vi "Run Command-Chris 1.9.vi"(2 "Line Index In":i32, 3 "Script":string) -> (0 "Line Index Out":i32, 1 "Done":bool)   [LabVIEW 2017, in "Apple script.lvlib"]
doc: "Looks at a line and runs the appropriate command. Add new commands to this vi."
uses:
  Apple script.lvlib
  Robot Global Data.vi
  <vilib>/addons/control/pid/pid.llb/PID.vi
  <vilib>/addons/control/pid/pid.llb/PID (DBL).vi
  Support Code/Angle Distance.vi
  Support Code/Pigeon Gyro.vi
  Support Code/Encoders.vi
  <vilib>/Rock Robotics/Network Tables/NT Write Value.vi
  <vilib>/Rock Robotics/Network Tables/NT Write Numeric Array.vi
  Timer.vi
  Parse Subcommand.vi
panel:
  in  "Error? 2":bool
  in  "Error?":bool
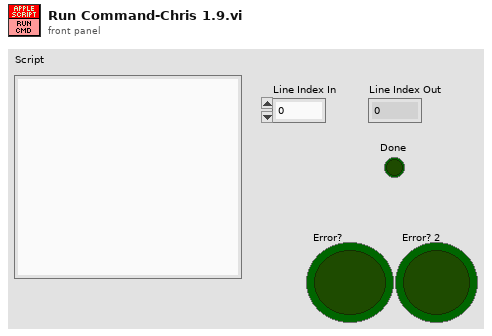
[diagram p1: front panel]
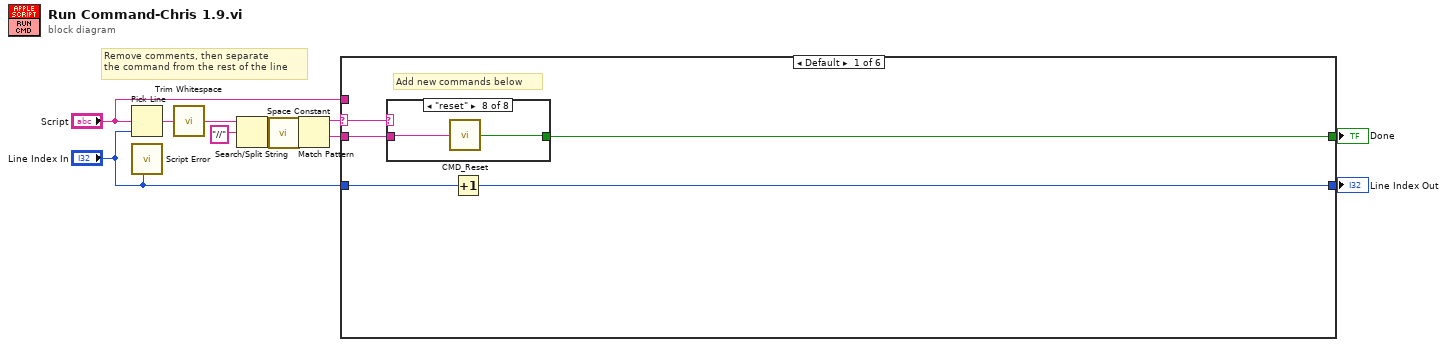
[diagram p0: block diagram]
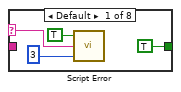
[diagram p2: hidden frame]
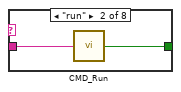
[diagram p3: hidden frame]
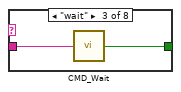
[diagram p4: hidden frame]
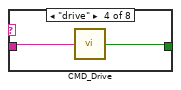
[diagram p5: hidden frame]
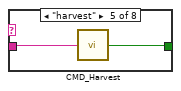
[diagram p6: hidden frame]
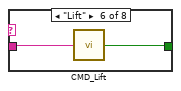
[diagram p7: hidden frame]
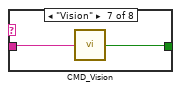
[diagram p8: hidden frame]
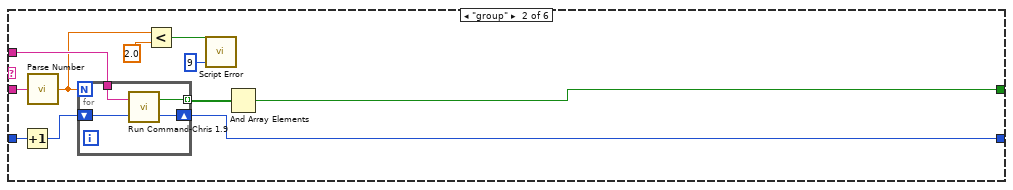
[diagram p9: hidden frame]
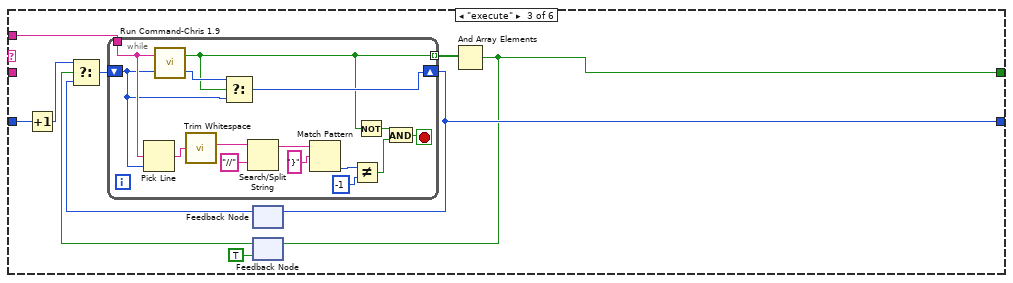
[diagram p10: hidden frame]
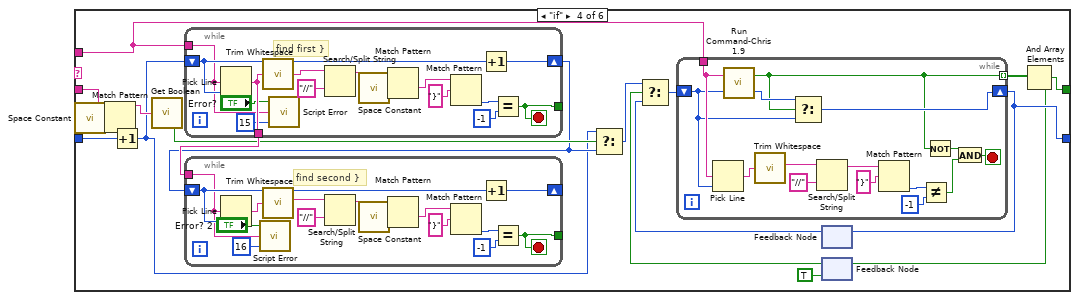
[diagram p11: hidden frame]
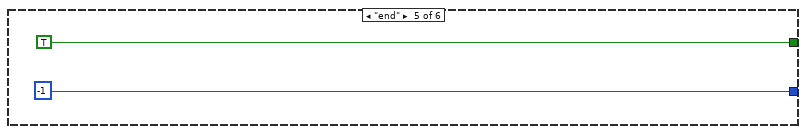
[diagram p12: hidden frame]
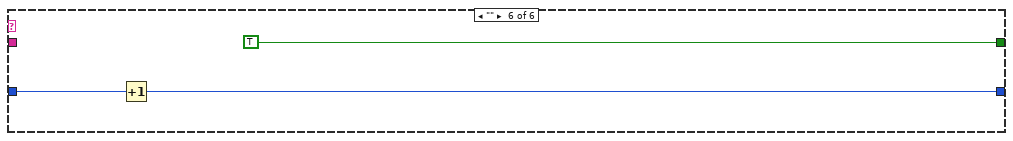
[diagram p13: hidden frame]
diagram:
  # "Remove comments, then separate\nthe command from the rest of the line"
  n1 = Pick Line(multi-line string="Script", line index="Line Index In") -> (output string=w8:string)  [unwired: 1 in]
  n2 = call "Script Error.vi"("Line Number"="Line Index In") -> ()  [unwired: 4 in, 1 out]
  n3 = call <vilib>:"Trim Whitespace.vi"("string"=w8) -> ("trimmed string"=w6:string)  [unwired: 1 in]
  n4 = Search/Split String(string=w6, search string/char (-)="//") -> (substring before match=w5:string)  [unwired: 1 in, 2 out]
  n5 = call <vilib>:"Space Constant.vi"() -> ("String"=w11:string)
  n6 = Match Pattern(string=w5, regular expression=w11) -> (before substring=w4:string, after substring=w3:string)  [unwired: 1 in, 2 out]
  n7 = case shown="Default" w4 {
    selector: w4 -> [w14 _ _ _ _ _]
    tunnel: "Script" -> [_ w45 w58 w83 _ _]
    tunnel: "Line Index In" -> [w16 w43 w59 w77 _ w140]
    tunnel: [w13 w35 w52 w81 TRUE ("Running") TRUE ("Running")] -> w2
    tunnel: [w15 w44 w53 w82 -1 ("Line Index Out") w139] -> w1
    tunnel: w3 -> [w12 w37 _ w78 _ _]
    frame Default {
      # "Add new commands below"
      n8 = case shown="\"reset\"" w14 {
        selector: w14 -> [w17 _ _ _ _ _ _ _]
        tunnel: [TRUE w21 w24 w25 w27 w29 w31 w33] -> w13
        tunnel: w12 -> [_ w22 w23 w26 w28 w30 w32 w34]
        frame Default {
          n9 = call "Script Error.vi"("Error?"=TRUE, "Error Details"=w17, "Error Code"=3) -> ()  [unwired: 2 in, 1 out]
        }
        frame "run" {
          n10 = call "CMD_Run.vi"("Line"=w22) -> ("Done"=w21:bool)
        }
        frame "wait" {
          n11 = call "CMD_Wait.vi"("Line"=w23) -> ("Done"=w24:bool)
        }
        frame "drive" {
          n12 = call "CMD_Drive.vi"("Line"=w26) -> ("Done"=w25:bool)
        }
        frame "harvest" {
          n13 = call "CMD_Harvest.vi"("Line"=w28) -> ("Done"=w27:bool)
        }
        frame "Lift" {
          n14 = call "CMD_Lift.vi"("Line"=w30) -> ("Done"=w29:bool)
        }
        frame "Vision" {
          n15 = call "CMD_Vision.vi"("Line"=w32) -> ("Done"=w31:bool)
        }
        frame "reset" {
          n16 = call "CMD_Reset.vi"("Line"=w34) -> ("Done"=w33:bool)
        }
      }
      n17 = Increment(x=w16) -> (x+1=w15:i32)
    }
    frame "group" {
      n18 = Increment(x=w43) -> (x+1=w42:i32)
      n19 = call "Parse Number.vi"("String"=w37) -> ("Number"=w40:dbl)
      n20 = for {
        N: w40 -> [_]
        tunnel: w45 -> [w49]
        tunnel: [w48] -> w36 mode=indexing
        shift-right: [w47] -> w44
        shift-left: w42 -> [w46]
        n21 = call "Run Command-Chris 1.9.vi"("Line Index In"=w46, "Script"=w49) -> ("Line Index Out"=w47:i32, "Done"=w48:bool)
      }
      n22 = Less?(x=w40, y=2.0) -> (x < y?=w39:bool)
      n23 = call "Script Error.vi"("Error?"=w39, "Error Code"=9) -> ()  [unwired: 3 in, 1 out]
      n24 = And Array Elements(Boolean array=w36) -> (logical AND=w35:bool)
    }
    frame "execute" {
      n25 = Increment(x=w59) -> (x+1=w55:i32)
      n26 = feedback #1() -> (w54:i32)  [unwired: 1 in]
      n27 = feedback #2(TRUE) -> (w51:bool)
      n28 = Select(t=w55, s=w51, f=w54) -> (s? t:f=w56:i32)
      n29 = while {
        tunnel: w58 -> [w68]
        tunnel: [w61] -> w57 mode=indexing
        shift-right: [w65] -> w53
        shift-left: w56 -> [w64]
        stop <- w60 stop-if-true
        n30 = Pick Line(multi-line string=w68, line index=w64) -> (output string=w70:string)  [unwired: 1 in]
        n31 = call "Run Command-Chris 1.9.vi"("Line Index In"=w64, "Script"=w68) -> ("Line Index Out"=w66:i32, "Done"=w61:bool)
        n32 = call <vilib>:"Trim Whitespace.vi"("string"=w70) -> ("trimmed string"=w71:string)  [unwired: 1 in]
        n33 = Select(t=w66, s=w61, f=w64) -> (s? t:f=w65:i32)
        n34 = Search/Split String(string=w71, search string/char (-)="//") -> (substring before match=w67:string)  [unwired: 1 in, 2 out]
        n35 = Match Pattern(string=w67, regular expression="}" ("search string/char (-)")) -> (offset past match=w73:i32)  [unwired: 1 in, 3 out]
        n36 = Not Equal?(x=w73, y=-1) -> (x != y?=w63:bool)
        n37 = Not(x=w61) -> (.not. x?=w62:bool)
        n38 = And(x=w62, y=w63) -> (x .and. y?=w60:bool)
      }
      n39 = feedback-in #1(w53) -> ()
      n40 = And Array Elements(Boolean array=w57) -> (logical AND=w52:bool)
      n41 = feedback-in #2(w52) -> ()
    }
    frame "if" {
      n42 = call <vilib>:"Space Constant.vi"() -> ("String"=w80:string)
      n43 = Match Pattern(string=w78, regular expression=w80) -> (before substring=w79:string)  [unwired: 1 in, 3 out]
      n44 = Increment(x=w77) -> (x+1=w76:i32)
      n45 = call "Get Boolean.vi"("Name"=w79) -> ("Value"=w90:bool)
      n46 = while {
        tunnel: w83 -> [w124]
        shift-right: [w128] -> w89
        shift-left: w76 -> [w129]
        tunnel: [w127] -> w91
        tunnel: [w126] -> _
        stop <- w126 stop-if-true
        # "find first }"
        n47 = Pick Line(multi-line string=w124, line index=w129) -> (output string=w127:string)  [unwired: 1 in]
        n48 = call <vilib>:"Trim Whitespace.vi"("string"=w127) -> ("trimmed string"=w125:string)  [unwired: 1 in]
        n49 = call "Script Error.vi"("Error?"="Error?", "Error Details"=w124, "Error Code"=15) -> ()  [unwired: 2 in, 1 out]
        n50 = Search/Split String(string=w125, search string/char (-)="//") -> (substring before match=w133:string)  [unwired: 1 in, 2 out]
        n51 = call <vilib>:"Space Constant.vi"() -> ("String"=w132:string)
        n52 = Match Pattern(string=w133, regular expression=w132) -> (after substring=w130:string)  [unwired: 1 in, 3 out]
        n53 = Match Pattern(string=w130, regular expression="}" ("search string/char (-)")) -> (offset past match=w135:i32)  [unwired: 1 in, 3 out]
        n54 = Increment(x=w129) -> (x+1=w128:i32)
        n55 = Equal?(x=w135, y=-1) -> (x = y?=w126:bool)
      }
      n56 = while {
        tunnel: w91 -> [w109]
        shift-right: [w111] -> _
        shift-left: w89 -> [w112]
        tunnel: [w110] -> _
        stop <- w110 stop-if-true
        # "find second }"
        n57 = Pick Line(multi-line string=w109, line index=w112) -> (output string=w116:string)  [unwired: 1 in]
        n58 = call "Script Error.vi"("Error?"="Error? 2", "Error Details"=w109, "Error Code"=16) -> ()  [unwired: 2 in, 1 out]
        n59 = call <vilib>:"Trim Whitespace.vi"("string"=w116) -> ("trimmed string"=w117:string)  [unwired: 1 in]
        n60 = Search/Split String(string=w117, search string/char (-)="//") -> (substring before match=w118:string)  [unwired: 1 in, 2 out]
        n61 = call <vilib>:"Space Constant.vi"() -> ("String"=w115:string)
        n62 = Match Pattern(string=w118, regular expression=w115) -> (after substring=w113:string)  [unwired: 1 in, 3 out]
        n63 = Match Pattern(string=w113, regular expression="}" ("search string/char (-)")) -> (offset past match=w120:i32)  [unwired: 1 in, 3 out]
        n64 = Increment(x=w112) -> (x+1=w111:i32)
        n65 = Equal?(x=w120, y=-1) -> (x = y?=w110:bool)
      }
      n66 = Select(t=w76, s=w90, f=w89) -> (s? t:f=w84:i32)
      n67 = feedback #3() -> (w86:i32)  [unwired: 1 in]
      n68 = feedback #4(TRUE) -> (w85:bool)
      n69 = Select(t=w84, s=w85, f=w86) -> (s? t:f=w87:i32)
      n70 = while {
        tunnel: w83 -> [w100]
        tunnel: [w93] -> w88 mode=indexing
        shift-right: [w97] -> w82
        shift-left: w87 -> [w96]
        stop <- w92 stop-if-true
        n71 = Pick Line(multi-line string=w100, line index=w96) -> (output string=w102:string)  [unwired: 1 in]
        n72 = call "Run Command-Chris 1.9.vi"("Line Index In"=w96, "Script"=w100) -> ("Line Index Out"=w98:i32, "Done"=w93:bool)
        n73 = call <vilib>:"Trim Whitespace.vi"("string"=w102) -> ("trimmed string"=w103:string)  [unwired: 1 in]
        n74 = Select(t=w98, s=w93, f=w96) -> (s? t:f=w97:i32)
        n75 = Search/Split String(string=w103, search string/char (-)="//") -> (substring before match=w99:string)  [unwired: 1 in, 2 out]
        n76 = Match Pattern(string=w99, regular expression="}" ("search string/char (-)")) -> (offset past match=w105:i32)  [unwired: 1 in, 3 out]
        n77 = Not Equal?(x=w105, y=-1) -> (x != y?=w95:bool)
        n78 = Not(x=w93) -> (.not. x?=w94:bool)
        n79 = And(x=w94, y=w95) -> (x .and. y?=w92:bool)
      }
      n80 = feedback-in #3(w82) -> ()
      n81 = And Array Elements(Boolean array=w88) -> (logical AND=w81:bool)
      n82 = feedback-in #4(w81) -> ()
    }
    frame "end" {
    }
    frame "" {
      n83 = Increment(x=w140) -> (x+1=w139:i32)
    }
  }
  "Line Index Out" <- w1
  "Done" <- w2
